vi "PT_Setup.vi"(11 "Actor's Event Messenger":refnum<class "EventMessenger.lvclass">) -> ()   [LabVIEW 2023]
uses:
  <vilib>/drjdpowell/Messenging/Core Messengers/EventMessenger/EventMessenger.lvclass
  <vilib>/drjdpowell/Messenging/Core Messages/Message/MSG.lvclass/MSG.ctl
  <vilib>/drjdpowell/Messenging/Core Messages/VarMessage/VariantMSG.lvclass/VariantMSG.ctl
  a6cb60a9-7e9f-4158-b971-5cd5afdacf86.vi
  a6cb60a9-7e9f-4158-b971-5cd5afdacf86.vi/afc9f7b6-782e-46b2-95da-8e576e84c933.vi
  <vilib>/drjdpowell/Messenging/Core Messages/VarMessage/Write VariantMSG.vi
  <vilib>/drjdpowell/Messenging/Core Messages/Message/Overwrite Reply Address.vi
  <vilib>/drjdpowell/Messenging/Core Messages/Message/Label Message.vi
  <vilib>/drjdpowell/Messenging/Core Messages/VarMessage/VariantMSG.lvclass
  C:/Program Files (x86)/National Instruments/LabVIEW 2023/vi.lib/drjdpowell/Messenging/Core Messages/Message/MSG.lvclass
  <vilib>/drjdpowell/Messenging/Core Messengers/Send/Send.lvclass
  <vilib>/drjdpowell/Messenging/Core Messages/Message/MSG.lvclass
panel:
  in  "Names":string[](array[string])=["PT 1", "PT 2", "PT 3", "PT 4"]
  in  "OK":bool
  in  "Offsets":dbl[](array[numeric])=[0.0, 0.0, 0.0, 0.0]
  in  "Multipliers":dbl[](array[numeric])=[1.0, 1.0, 1.0, 1.0]
  out "Channels":string[](array[string])=["AIN0", "AIN2", "AIN4", "AIN6"]
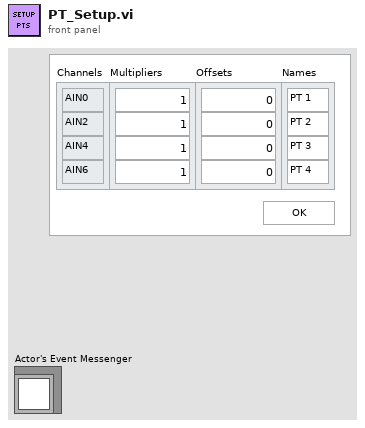
[diagram p1: front panel]
types:
  T1 = cluster{"Multipliers":dbl[], "Offsets":dbl[], "Names":string[]}
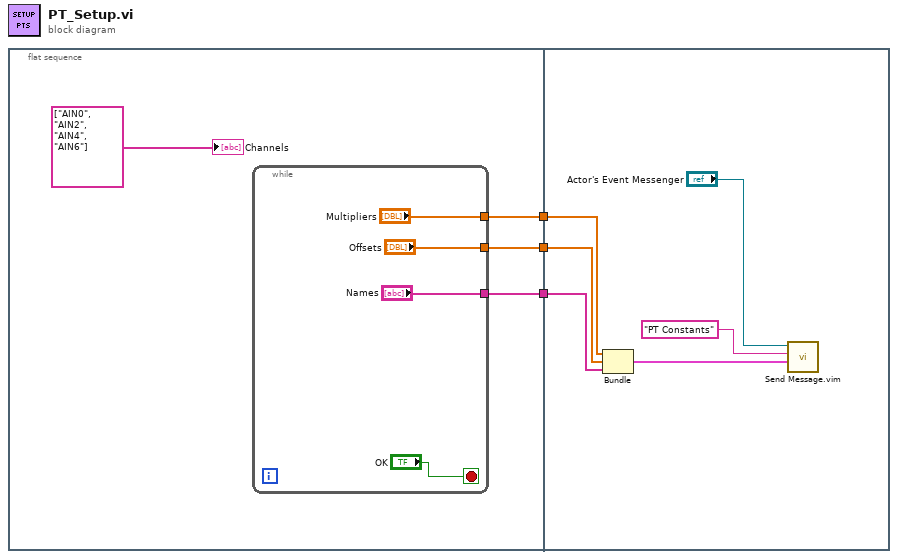
[diagram p0: block diagram]
diagram:
  n1 = flat-sequence {
    tunnel: [w6] -> w3
    tunnel: [w5] -> w2
    tunnel: [w4] -> w1
    tunnel: w3 -> [w14]
    tunnel: w2 -> [w15]
    tunnel: w1 -> [w12]
    frame #0 {
      n2 = while {
        tunnel: ["Multipliers"] -> w5
        tunnel: ["Offsets"] -> w6
        tunnel: ["Names"] -> w4
        stop <- "OK" stop-if-true
      }
      "Channels" <- string[] ["AIN0", "AIN2", "AIN4", "AIN6"] ("Channels")
    }
    frame #1 {
      n3 = Bundle("Multipliers"=w15, "Offsets"=w14, "Names"=w12) -> (w13:T1)  [unwired: 1 in]
      n4 = call "Send Message.vim"("Contents"=w13, "Label or Message"="PT Constants", "Address"="Actor's Event Messenger") -> ()  [unwired: 7 in, 2 out]
    }
  }
